vi "save ini configuration to image file path.vi"   [LabVIEW 2012]
uses:
  GFG/GFGpathGet.vi
  GFG/GFG library.lvlib
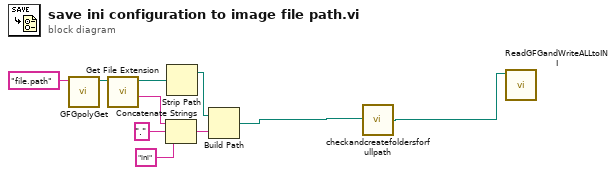
[diagram p0: block diagram]
diagram:
  n1 = call-poly "GFGpolyGet.vi"("Variable Name in"="file.path") -> ("Path"=w6:path)  [unwired: 9 in, 1 out]
  n2 = call <vilib>:"Get File Extension.vi"("file"=w6) -> ("filename without extension"=w7:string)  [unwired: 7 in, 3 out]
  n3 = Concatenate Strings(w7, "." ("string"), "ini" ("string")) -> (w9:string)
  n4 = Strip Path(path=w6) -> (stripped path=w8:path)  [unwired: 1 out]
  n5 = Build Path(base path=w8, name or relative path=w9) -> (appended path=w2:path)
  n6 = call "checkandcreatefoldersforfullpath.vi"("Path IN"=w2) -> ("Path OUT"=w1:path)  [unwired: 4 in]
  n7 = call "ReadGFGandWriteALLtoINI.vi"("Path"=w1) -> ()  [unwired: 10 in, 1 out]
